vi "Lester Roche y Elmin Mejia Prueba 2 corregida.vi"() -> ()   [LabVIEW 2011]
panel:
  out "Mayor a 40":bool
  out "Contador >40":dbl
  out "Temperatura Promedio":dbl
  out "Temperatura Menor":dbl
  out "Temperatura mayor":dbl
  out "temperatura":i32(slide) scale=0.0..60.0
  # "Se tiene que generar una temperatura entre 1-60, luego debera de encender un \nled cada vez, que la temperatura sea mayor a 40 y debera de contarla.\nSe tiene que obtener el numero mayor y menor.\nLa temperatura promedio solo se obtiene de las temperatura mayores a 30. \nHacerlo 5 veces, usar el ciclo for."
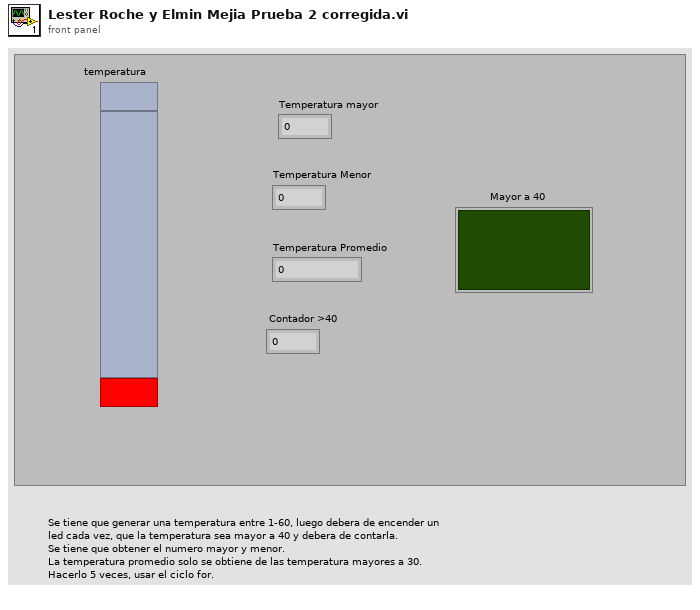
[diagram p1: front panel]
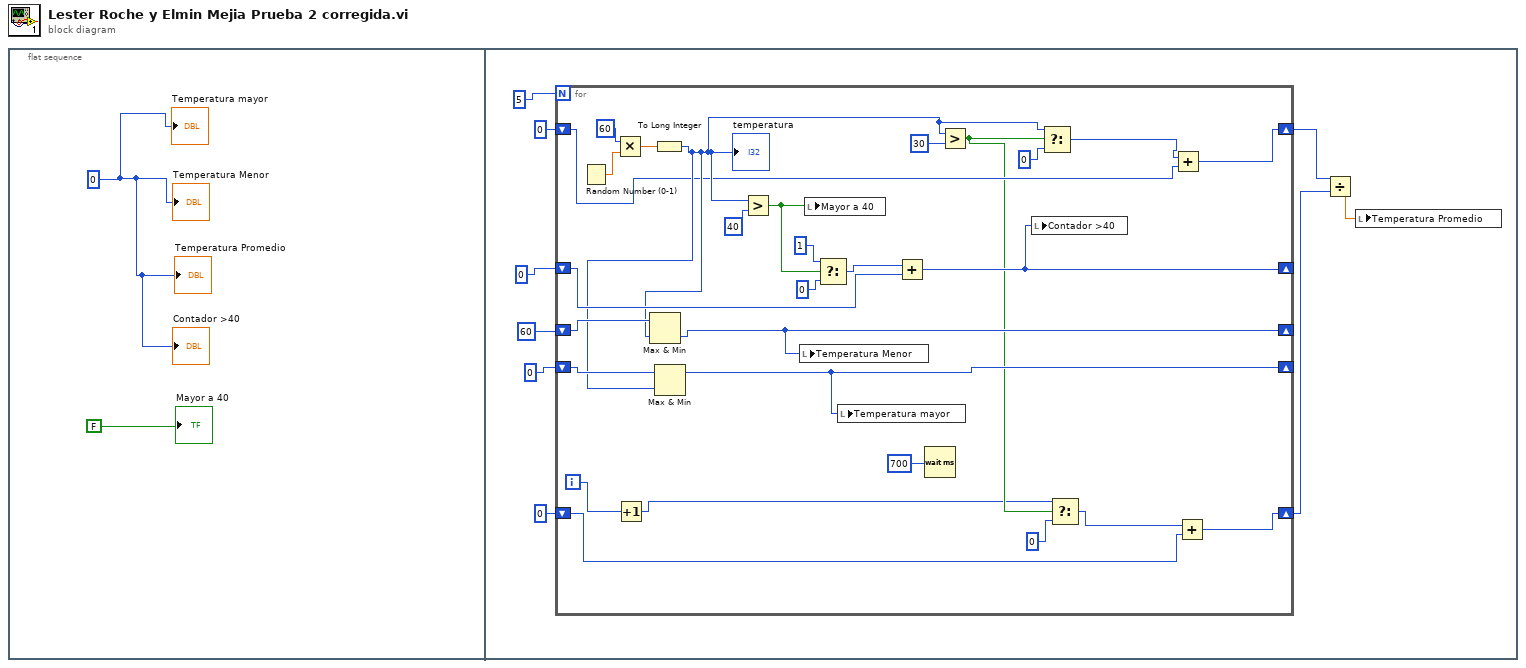
[diagram p0: block diagram]
diagram:
  n1 = flat-sequence {
    frame #0 {
      w1 = 0
      "Temperatura Promedio" <- w1
      "Contador >40" <- w1
      "Temperatura mayor" <- w1
      "Temperatura Menor" <- w1
      "Mayor a 40" <- FALSE
    }
    frame #1 {
      n2 = for {
        N: 5 -> [_]
        shift-right: [w33] -> _
        shift-left: 60 -> [w34]
        shift-right: [w31] -> _
        shift-left: 0 -> [w32]
        shift-right: [w24] -> _
        shift-left: 0 -> [w25]
        shift-right: [w19] -> w5
        shift-left: 0 -> [w18]
        shift-right: [w12] -> w4
        shift-left: 0 -> [w13]
        i -> [w30]
        n3 = Random Number (0-1)() -> (number: 0 to 1=w38:dbl)
        n4 = Multiply(x=60, y=w38) -> (x*y=w37:dbl)
        n5 = Increment(x=w30) -> (x+1=w16:i32)
        n6 = To Long Integer(number=w37) -> (32bit integer=w21:i32)
        "temperatura" <- w21
        n7 = Max & Min(x=w34, y=w21) -> (min(x,y)=w33:i32)  [unwired: 1 out]
        n8 = Max & Min(x=w32, y=w21) -> (max(x,y)=w31:i32)  [unwired: 1 out]
        n9 = Greater?(x=w21, y=40) -> (0:w35:bool)
        n10 = local write "Temperatura Menor"(w33) -> ()
        n11 = local write "Mayor a 40"(w35) -> ()
        n12 = Select(t=1, s=w35, f=0) -> (s? t:f=w26:i32)
        n13 = local write "Temperatura mayor"(w31) -> ()
        n14 = Add(x=w26, y=w25) -> (x+y=w24:i32)
        n15 = Wait (ms)(milliseconds to wait=700) -> ()  [unwired: 1 out]
        n16 = Greater?(x=w21, y=30) -> (0:w17:bool)
        n17 = local write "Contador >40"(w24) -> ()
        n18 = Select(t=w21, s=w17, f=0) -> (s? t:f=w20:i32)
        n19 = Select(t=w16, s=w17, f=0) -> (s? t:f=w14:i32)
        n20 = Add(x=w20, y=w18) -> (x+y=w19:i32)
        n21 = Add(x=w14, y=w13) -> (x+y=w12:i32)
      }
      n22 = Divide(x=w5, y=w4) -> (x/y=w7:dbl)
      n23 = local write "Temperatura Promedio"(w7) -> ()
    }
  }
